vi "Save Decoration Info.vi"(8 "error in":errorcluster, 10 "control info":T1[](array[typedef]) {"Decoration Level" items=["N/A", "Primary", "Secondary", "Tertiary", "Error", "Primary Fixed", "Secondary Fixed", "Tertiary Fixed", "Label Only", "No Change"]}, 11 "map in":map{string, refnum<vi>}(c390)) -> (0 "error out":errorcluster)   [LabVIEW 2021]
doc: "This VI will save all of the updated tag data for the decorations in the VI reference.\n\n<b>Code Developed By:</b>\nTechnology Service Corporation\nwww.tsc.com/atcs\n\nDeveloper:\nDaniel Coons"
uses:
  Material SubVIs/Material SubVIs.lvlib
  decorations info--typedef.ctl
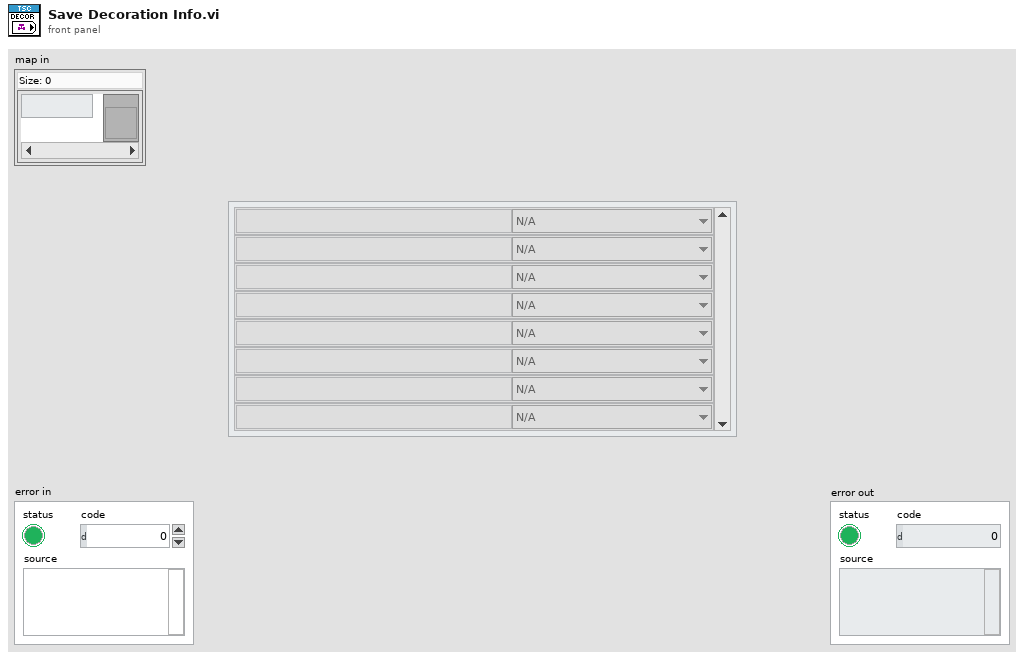
[diagram p1: front panel]
types:
  T1 = typedef "decorations info--typedef.ctl" = cluster{"label":string, "Decoration Level":u16}
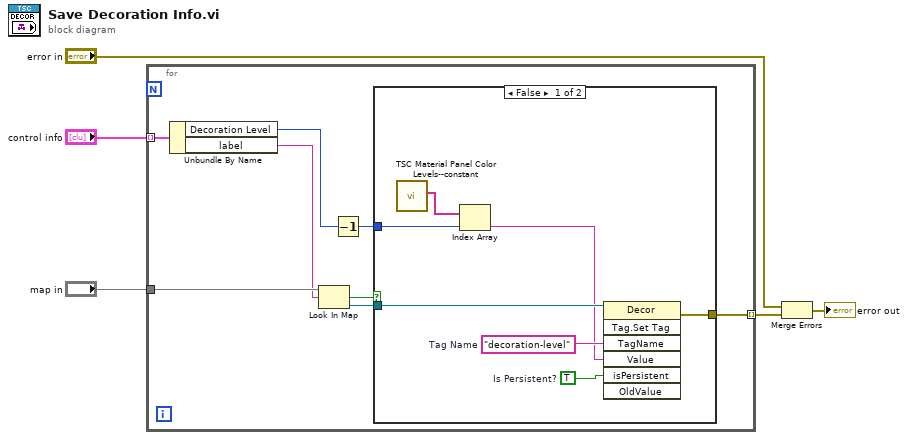
[diagram p0: block diagram]
diagram:
  n1 = for {
    tunnel: "map in" -> [w13]
    tunnel: "control info" -> [w12] mode=indexing
    tunnel: [w7] -> w3 mode=indexing
    n2 = Unbundle By Name(w12) -> ("Decoration Level"=w8:u16, "label"=w11:string)
    n3 = Look In Map(map=w13, key=w11) -> (key not found?=w10:bool, value=w9:refnum<vi>)  [unwired: 1 in]
    n4 = Decrement(x=w8) -> (x-1=w6:u16)
    n5 = case shown="False" w10 {
      tunnel: w9 -> [w16 _]
      tunnel: w6 -> [w19 _]
      tunnel: [w14 _] -> w7
      frame False {
        w17 = TRUE  # Is Persistent?
        w18 = "decoration-level"  # Tag Name
        n6 = call "TSC Material Panel Color Levels--constant.vi"() -> ("front panel color levels"=w20:string[])  [unwired: 11 in]
        n7 = Index Array(array=w20, index=w19) -> (element=w15:string)
        n8 = invoke class="Decor" method="Tag.Set Tag"(reference=w16, "TagName"=w18, "Value"=w15, "isPersistent"=w17) -> (error out=w14:errorcluster)  [unwired: 3 in, 6 out]
      }
      frame True {
      }
    }
  }
  n9 = Merge Errors("error in", w3) -> (→"error out":errorcluster)
